vi "Compare_all_VIs_library_llb.vi"() -> ()   [LabVIEW 2022 SP3]
panel:
  out "error out":errorcluster
  out "Same?":bool
  in  "Current VI":path
  # "Run thi vi from the project C:\\Users\\inigo\\Documents\\Kbiosystems\\LabVIEW Utilities\\compare VIs.lvproj\nrunnign outside the project does not launch the labview compare tool in interactive mode"
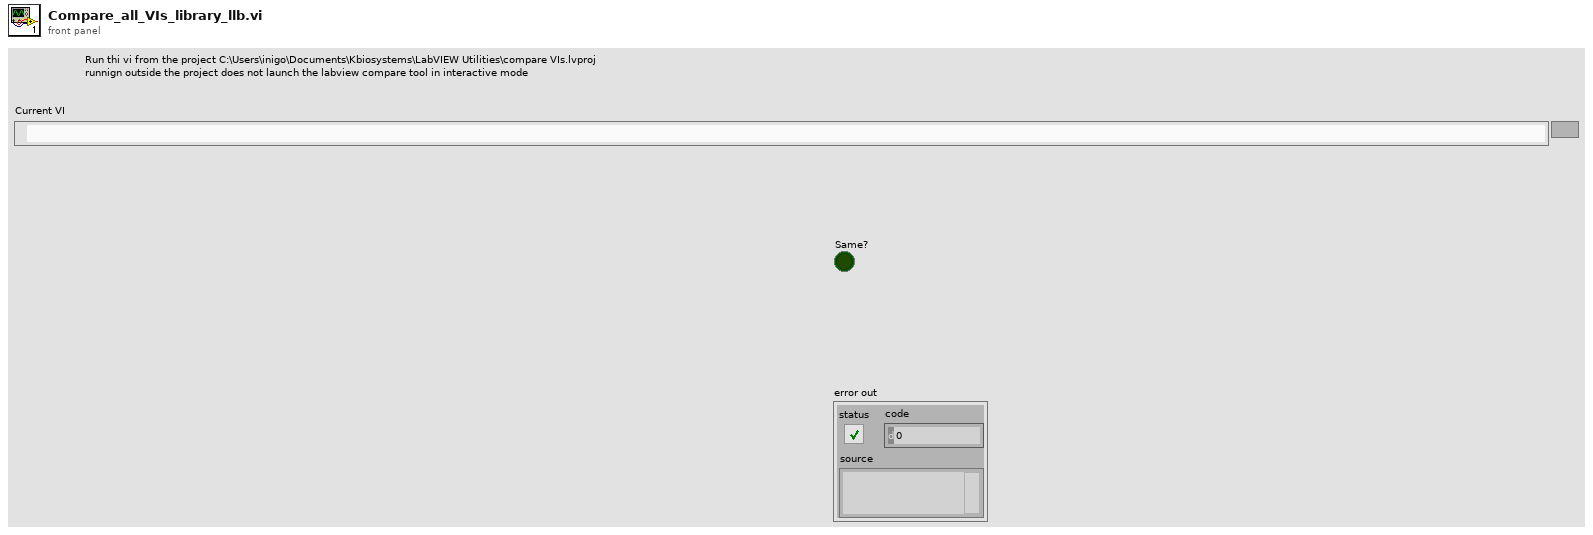
[diagram p1: front panel]
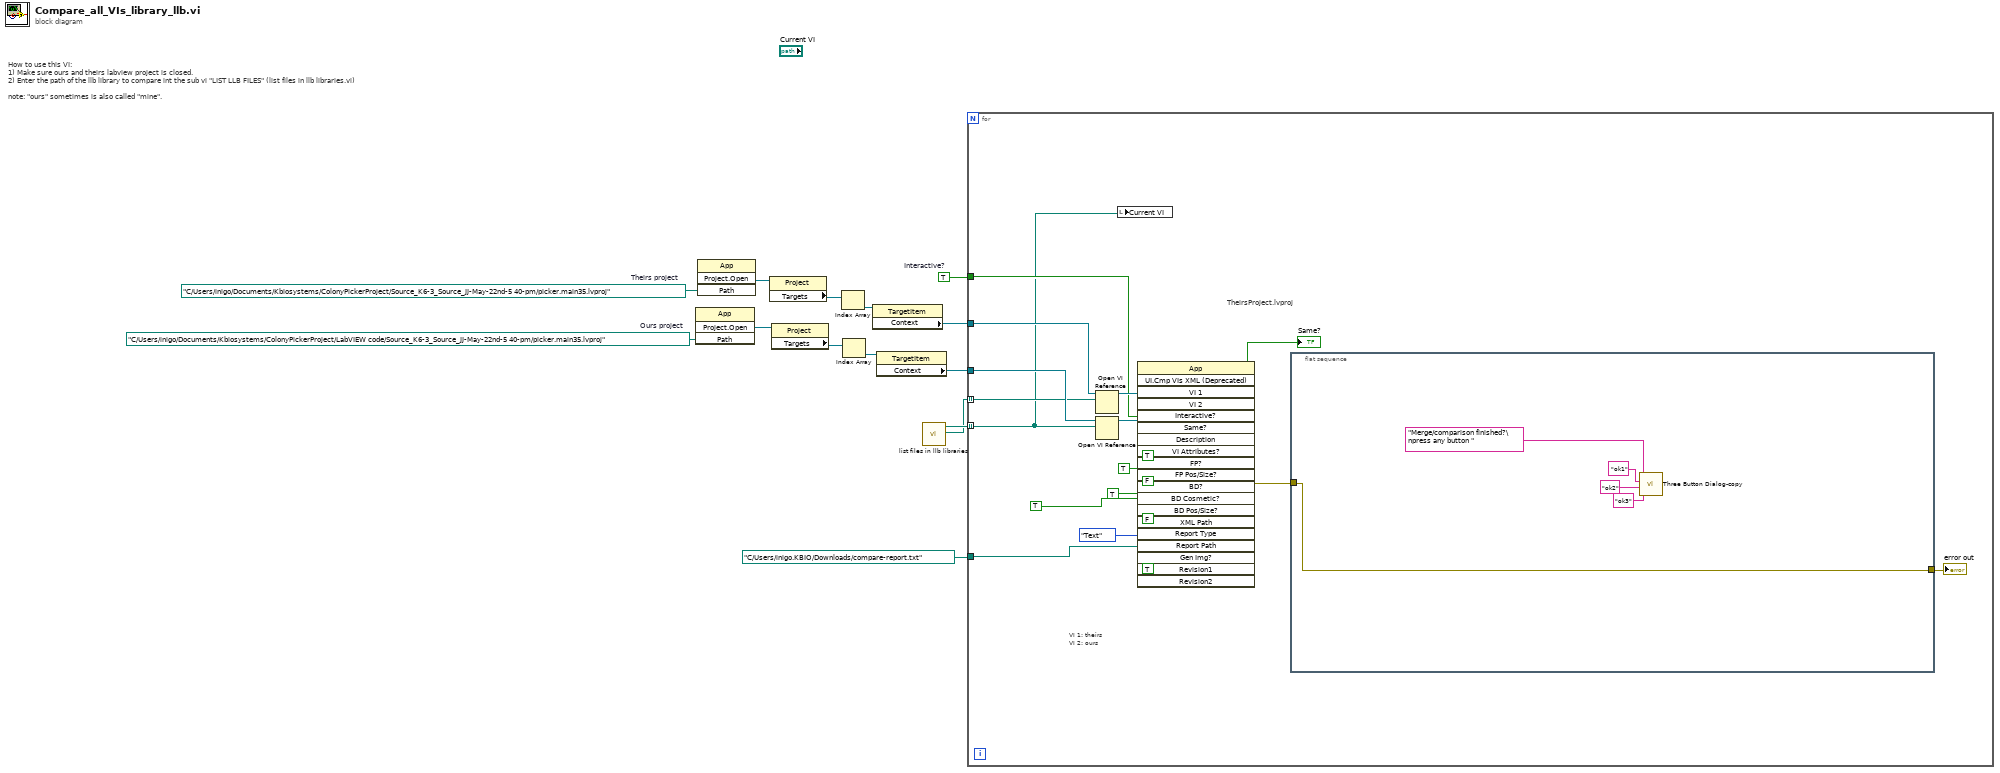
[diagram p0: block diagram]
diagram:
  w4 = TRUE  # Interactive?
  w14 = path "C:/Users/inigo/Documents/Kbiosystems/ColonyPickerProject/LabVIEW code/Source_K6-3_Source_JJ-May-22nd-5 40-pm/picker.main35.lvproj"  # Ours project
  w3 = path "C:/Users/inigo/Documents/Kbiosystems/ColonyPickerProject/Source_K6-3_Source_JJ-May-22nd-5 40-pm/picker.main35.lvproj"  # Theirs project
  # "How to use this VI:\n1) Make sure ours and theirs labview project is closed.\n2) Enter the path of the llb library to compare int the sub vi \"LIST LLB FILES\" (list files in llb libraries.vi)\n\nnote: \"ours\" sometimes is also called \"mine\"."
  n1 = invoke class="App" method="Project.Open"("Path"=w14) -> ("Project:Open"=w10:refnum<vi>)  [unwired: 3 in, 3 out]
  n2 = invoke class="App" method="Project.Open"("Path"=w3) -> ("Project:Open"=w13:refnum<vi>)  [unwired: 3 in, 3 out]
  n3 = property class="Project"(reference=w13) -> ("Targets"=w12:refnum<vi>[])  [unwired: 1 in, 2 out]
  n4 = property class="Project"(reference=w10) -> ("Targets"=w11:refnum<vi>[])  [unwired: 1 in, 2 out]
  n5 = Index Array(array=w12) -> (element=w9:refnum<vi>)  [unwired: 1 in]
  n6 = Index Array(array=w11) -> (element=w8:refnum<vi>)  [unwired: 1 in]
  n7 = property class="TargetItem"(reference=w9) -> ("Context"=w7:refnum<vi>)  [unwired: 1 in, 2 out]
  n8 = property class="TargetItem"(reference=w8) -> ("Context"=w6:refnum<vi>)  [unwired: 1 in, 2 out]
  n9 = call "list files in llb libraries.vi"() -> ("theirs"=w1:path[], "ours"=w2:path[])  [unwired: 10 in]
  n10 = for {
    tunnel: w7 -> [w27]
    tunnel: w6 -> [w26]
    tunnel: w4 -> [w18]
    tunnel: path "C:/Users/inigo.KBIO/Downloads/compare-report.txt" ("Result JSON Path") -> [w17]
    tunnel: w2 -> [w15] mode=indexing
    tunnel: w1 -> [w16] mode=indexing
    # "VI 1: theirs\nVI 2: ours"
    # "TheirsProject.lvproj"
    n11 = Open VI Reference(application reference (local)=w27, vi path=w16) -> (vi reference=w32:refnum<vi>)  [unwired: 4 in, 1 out]
    n12 = Open VI Reference(application reference (local)=w26, vi path=w15) -> (vi reference=w31:refnum<vi>)  [unwired: 4 in, 1 out]
    n13 = local write "Current VI"(w15) -> ()
    n14 = invoke class="App" method="UI.Cmp VIs XML (Deprecated)"("VI 1"=w32, "VI 2"=w31, "Interactive?"=w18, "VI Attributes?"=TRUE, "FP?"=TRUE, "FP Pos/Size?"=FALSE, "BD?"=TRUE, "BD Cosmetic?"=TRUE, "BD Pos/Size?"=FALSE, "Report Type"=enum32{"None", "Webpage", "Text", "MS Word"}."Text", "Report Path"=w17, "Gen Img?"=TRUE) -> (error out=w21:errorcluster, "Same?"=→"Same?":bool)  [unwired: 8 in, 18 out]
    n15 = flat-sequence {
      tunnel: w21 -> [w38]
      tunnel: [w38] -> w33
      frame #0 {
        n16 = call "Three Button Dialog-copy.vi"("Right Button Text (\"Cancel\")"="ok3" ("Right Button Text (\"Cancel\")"), "Center Button Text (\"No\")"="ok2" ("Center Button Text (\"No\")"), "Left Button Text (\"Yes\")"="ok1" ("Left Button Text (\"Yes\")"), "message"="Merge/comparison finished?\npress any button " ("Message")) -> ()  [unwired: 7 in, 1 out]
      }
    }
    "error out" <- w33
  }
